vi "Scan Setup.vi"(8 "error in (no error)":errorcluster, 11 "LCD Retarder in":refnum<class "LCD Retarder.lvclass">) -> (0 "error out":errorcluster, 1 "User Cancelled?":bool, 3 "LCD Retarder out":refnum<class "LCD Retarder.lvclass">)   [LabVIEW 2009, in "LCD Retarder.lvclass"]
uses:
  LCD Retarder.lvclass
  Utility Classes/Readable/Readable.lvclass
  LCD Retarder.lvclass/LCD Retarder.ctl
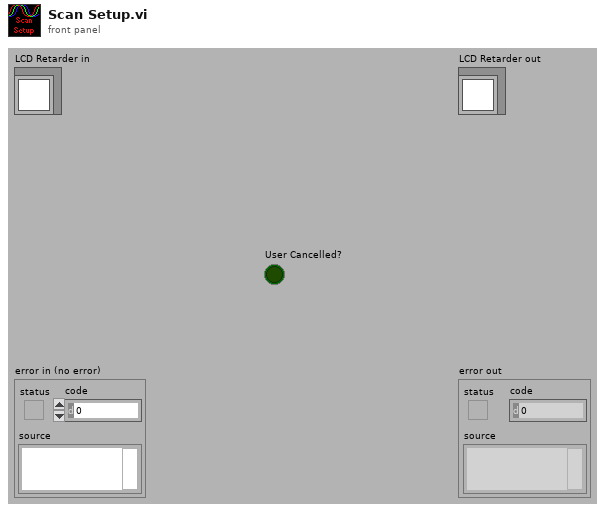
[diagram p1: front panel]
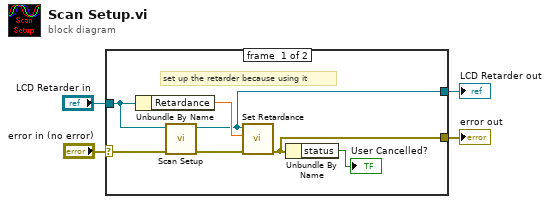
[diagram p0: block diagram]
diagram:
  n1 = case shown="No Error" "error in (no error)" {
    selector: "error in (no error)" -> [w7 w13]
    tunnel: "LCD Retarder in" -> [w9 w12]
    tunnel: [w8 w13] -> w3
    tunnel: [w5 w12] -> w1
    frame #0 {
      # "set up the retarder because using it"
      n2 = Unbundle By Name(w9) -> ("Retardance"=w6:dbl[unit])
      n3 = call-parent "Scan Setup.vi"("error in (no error)"=w7, "Instrument in"=w9) -> ("error out"=w11:errorcluster, "Instrument out"=w5:refnum<class "LCD Retarder.lvclass">)  [unwired: 8 out]
      n4 = call "Set Retardance.vi"("errorIN"=w11, "Retardance"=w6, "LCD in"=w5) -> ("errorOUT"=w8:errorcluster)  [unwired: 8 out]
      n5 = Unbundle By Name(w8) -> ("status"=→"User Cancelled?":bool)
    }
    frame #1 {
    }
  }
  "error out" <- w3
  "LCD Retarder out" <- w1
